vi "Schedule.EditFormula.vi"(8 "error in (no error)":errorcluster, 10 "Settings":string, 11 "ObjectSettings in":refnum<class "ObjectSettings.lvclass">) -> (0 "error out":errorcluster, 2 "Settings Out":string, 3 "ObjectSettings out":refnum<class "ObjectSettings.lvclass">)   [LabVIEW 2019, in "ObjectSettings.lvclass"]
uses:
  ObjectSettings.lvclass
  <vilib>/gmath/NI_Gmath.lvlib
  subVIs/typedefs/Schedule Types/Schedule--Formula.ctl
panel:
  in  "Resolution (nm)":dbl caption="Numeric"
  in  "OK":bool
  in  "Length (nm)":dbl caption="Numeric"
  out "XY Graph":cluster{"X Values":dbl[], "Y Values":dbl[]}(graph)
  in  "Formula":string
  out "Parse Error":bool
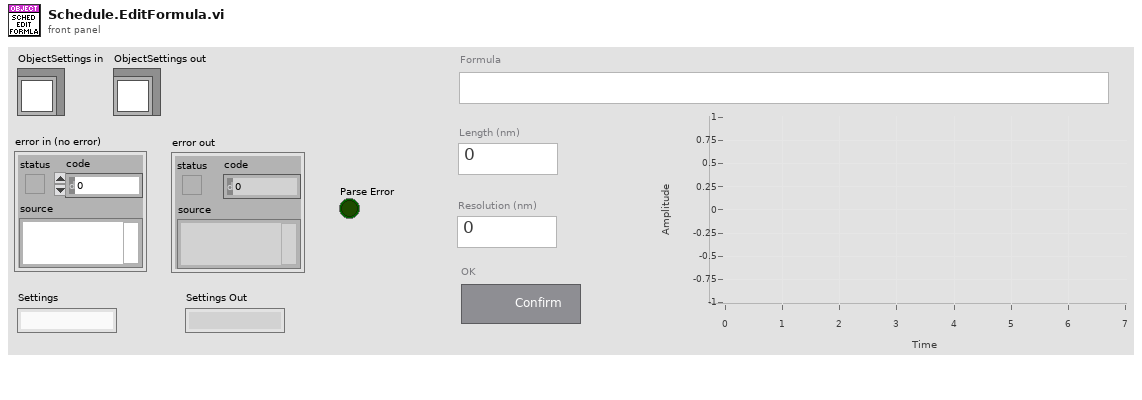
[diagram p1: front panel]
types:
  T1 = enum32{"Invalid", "Standard", "Closed", "Hidden", "Minimized", "Maximized"}
  T2 = enum32{"invalid app kind", "Development System", "Run Time System", "Student Edition", "Embedded LabVIEW", "Evaluation", "Custom"}
  T3 = typedef "Schedule--Formula.ctl" = cluster{"formula":string, "formula length (nm)":dbl, "formula resolution (nm)":dbl}
  T4 = cluster{"Core":cluster{"Current VI Reference":refnum<vi>, "Close Panel on Exit?":bool}, "ObjectSettings":refnum<class "ObjectSettings.lvclass">, "Formula":string, "Length (nm)":dbl, "Resolution (nm)":dbl, "Settings":string}
  T5 = cluster{"Current VI Reference":refnum<vi>, "Close Panel on Exit?":bool}
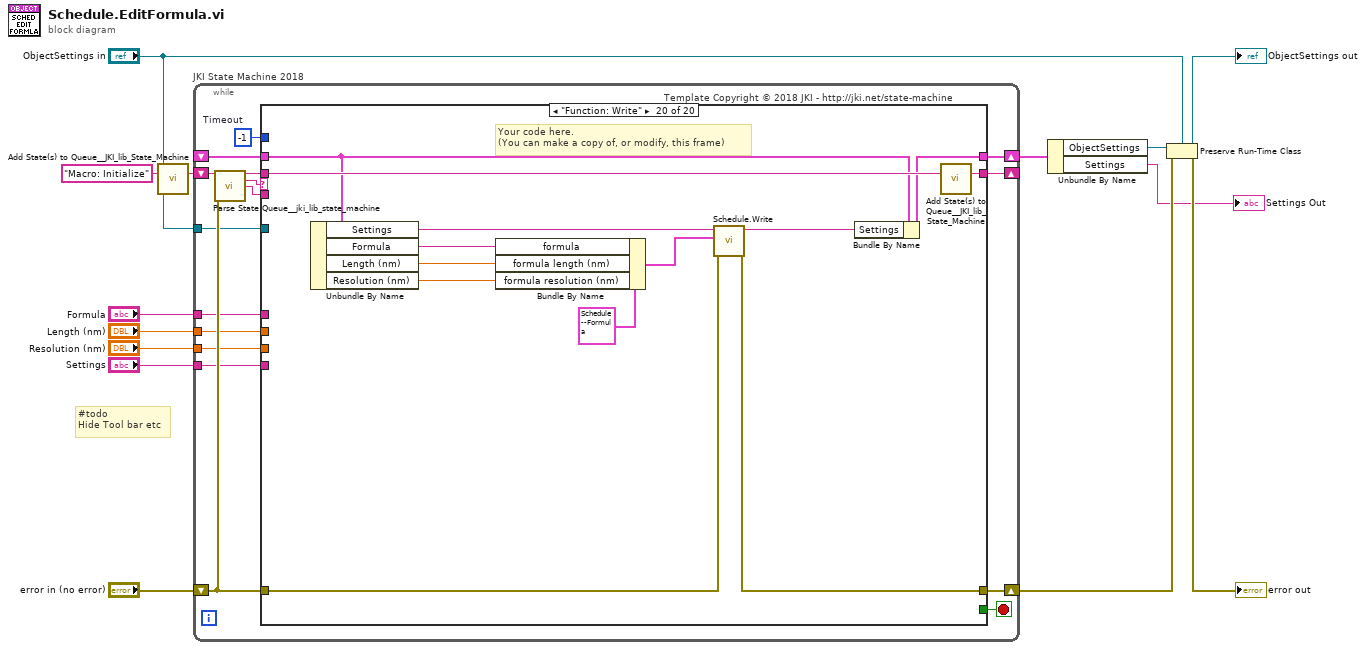
[diagram p0: block diagram]
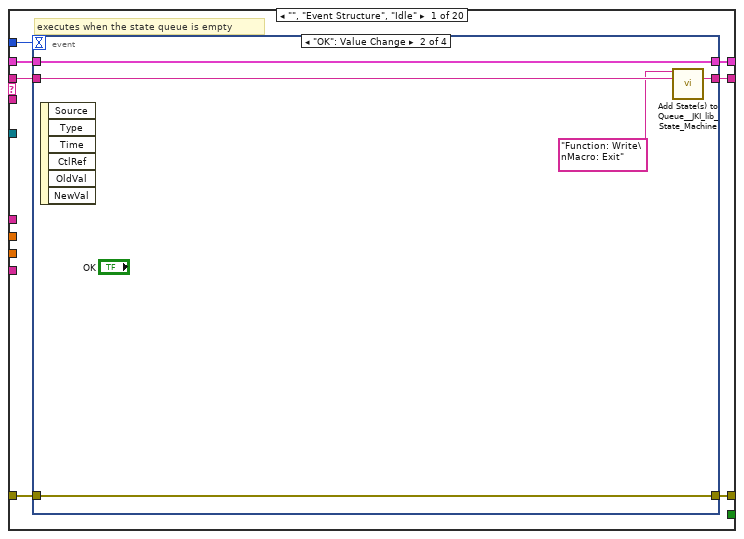
[diagram p2: hidden frame]
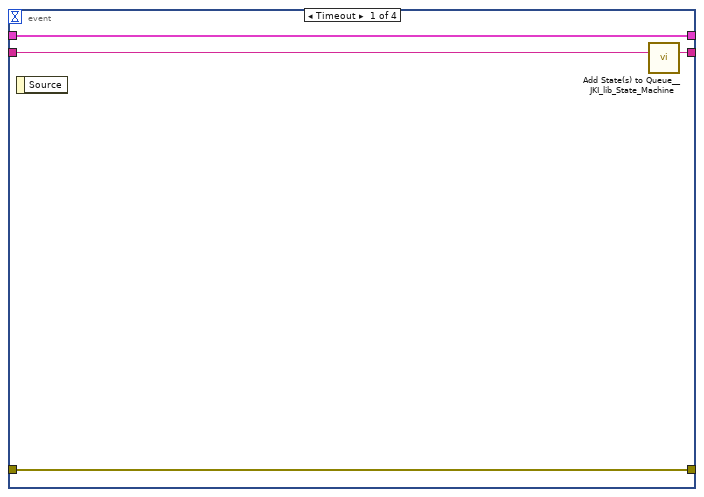
[diagram p3: hidden frame]
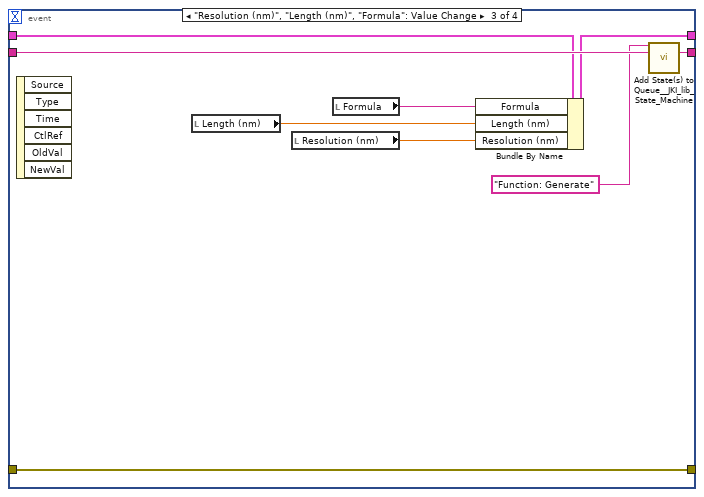
[diagram p4: hidden frame]
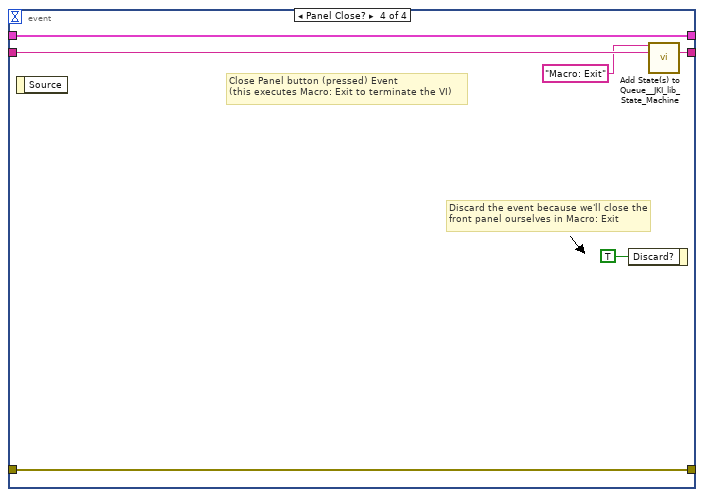
[diagram p5: hidden frame]
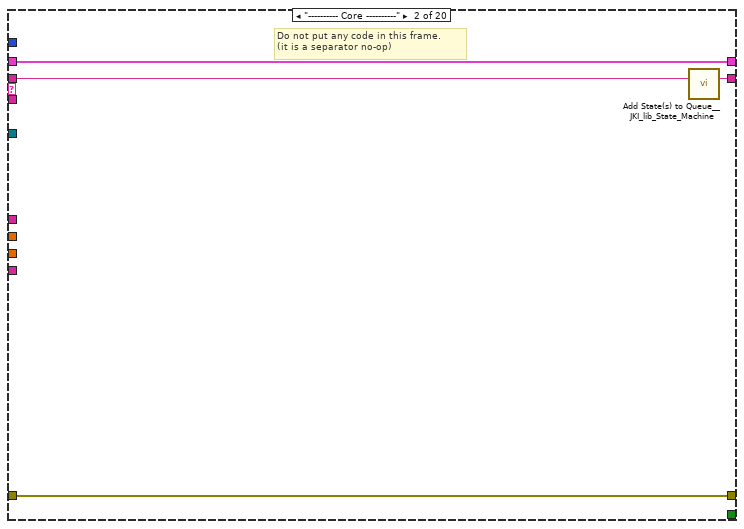
[diagram p6: hidden frame]
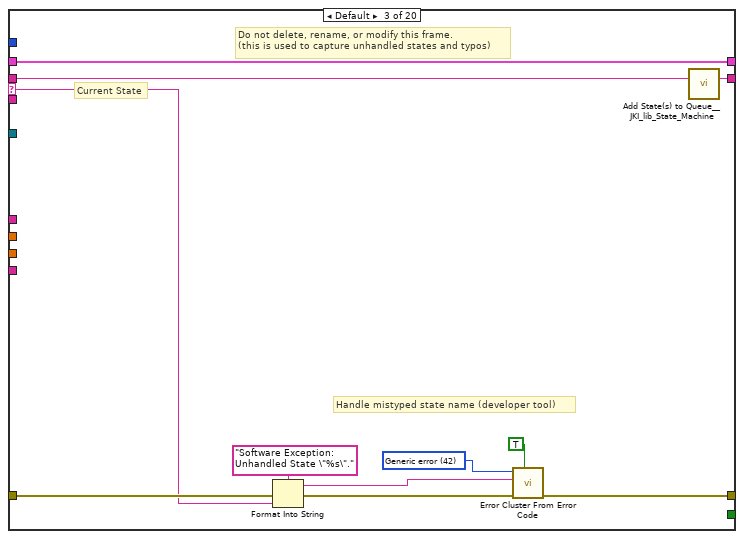
[diagram p7: hidden frame]
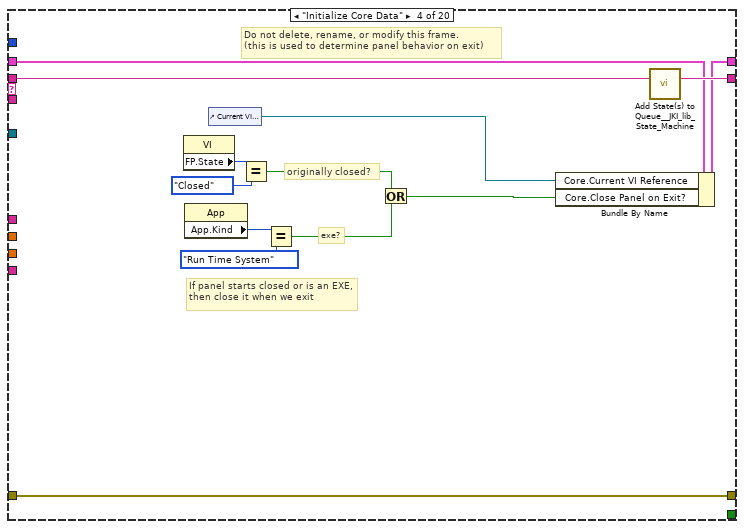
[diagram p8: hidden frame]
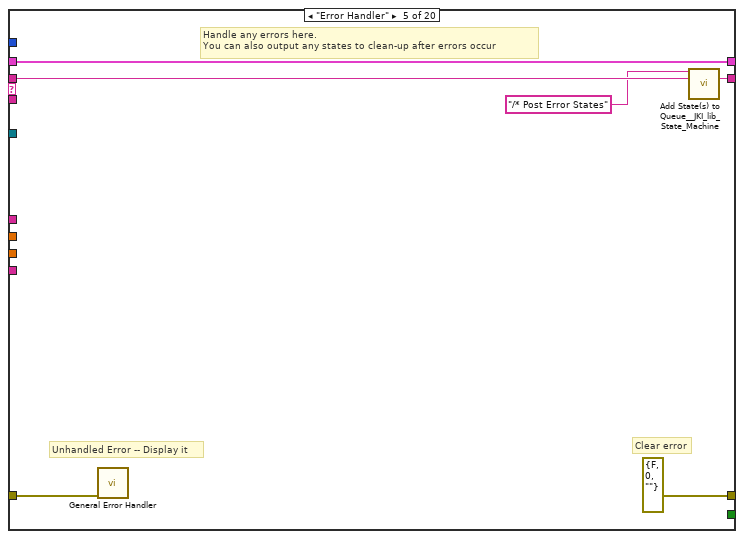
[diagram p9: hidden frame]
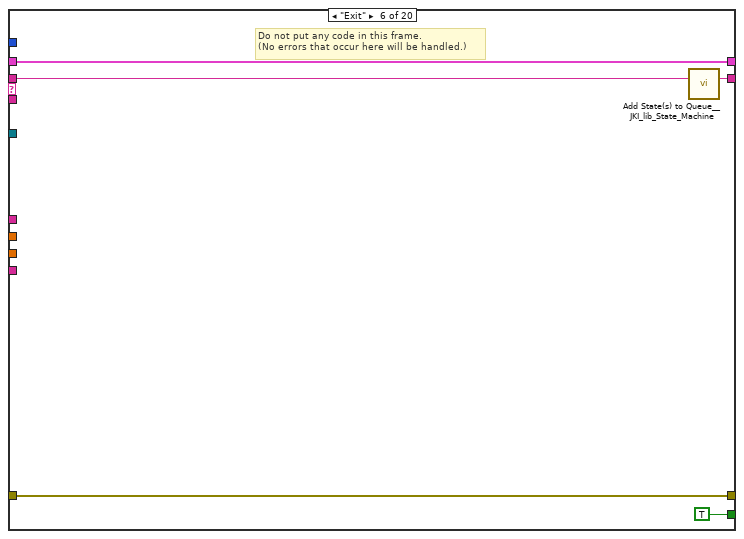
[diagram p10: hidden frame]
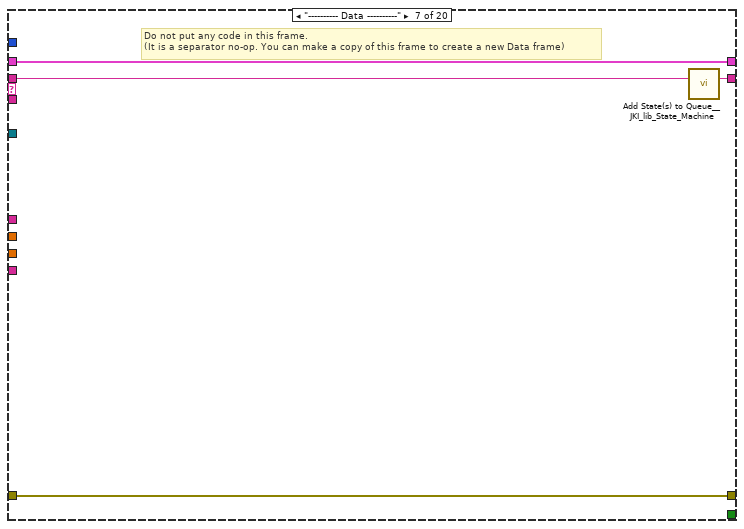
[diagram p11: hidden frame]
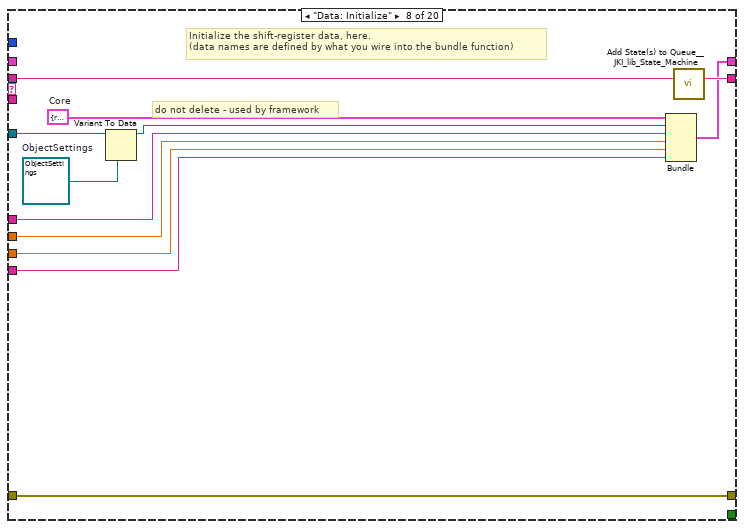
[diagram p12: hidden frame]
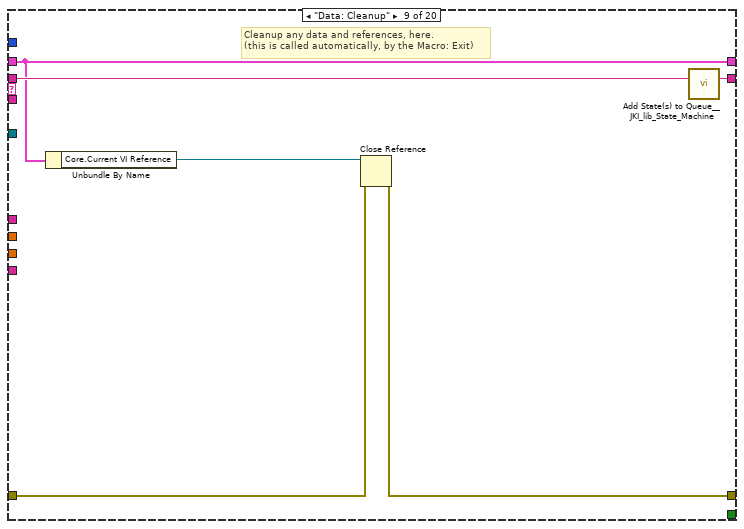
[diagram p13: hidden frame]
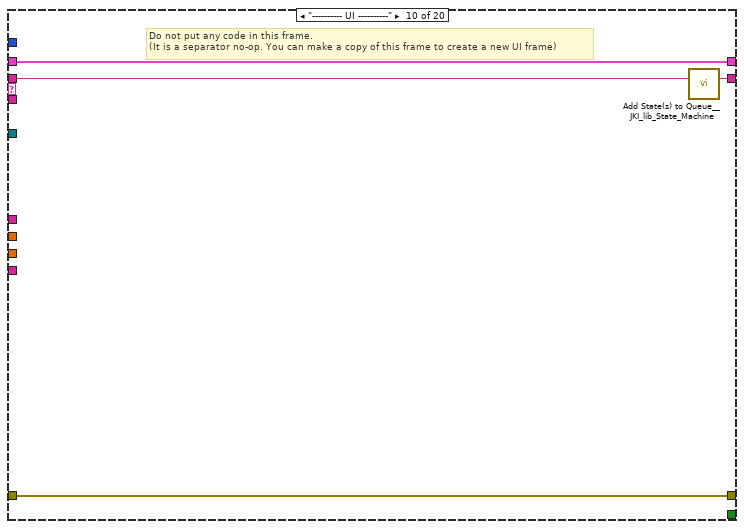
[diagram p14: hidden frame]
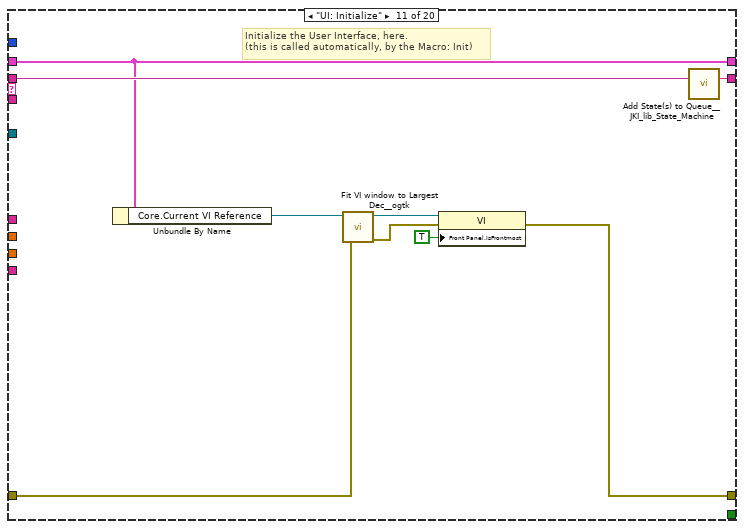
[diagram p15: hidden frame]
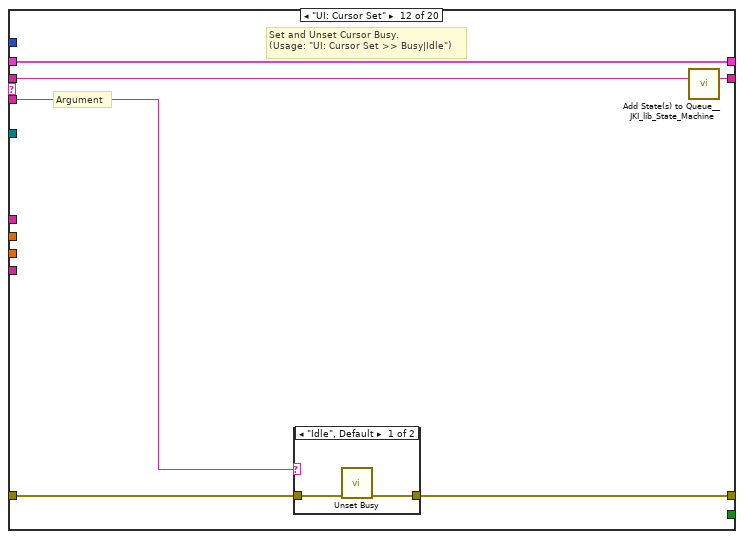
[diagram p16: hidden frame]
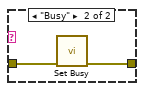
[diagram p17: hidden frame]
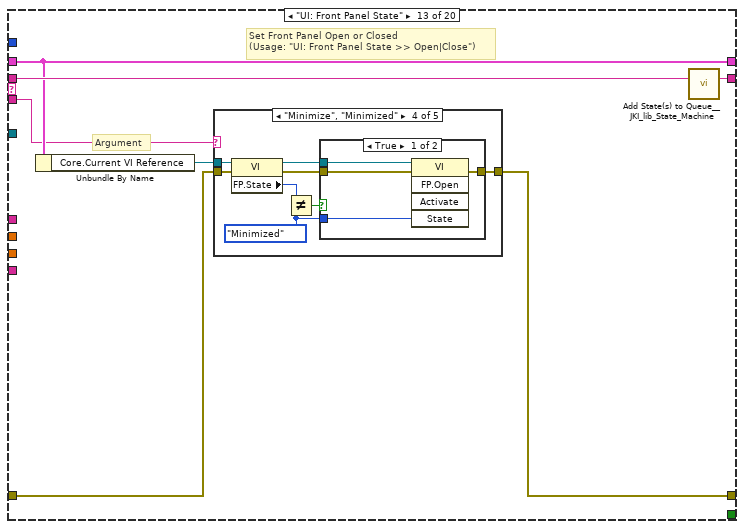
[diagram p18: hidden frame]
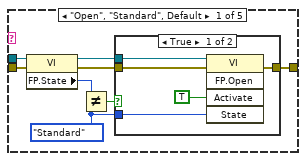
[diagram p19: hidden frame]
diagram:
  # "#todo\nHide Tool bar etc"
  n1 = call <vilib>:"Add State(s) to Queue__JKI_lib_State_Machine.vi"("State(s) in (\"\")"="Macro: Initialize") -> ("States Out"=w14:string)  [unwired: 14 in]
  n2 = while "JKI State Machine 2018" {
    shift-right: [w23] -> w12
    shift-left: _ -> [w22]
    shift-right: [w26] -> w7
    shift-left: "error in (no error)" -> [w20]
    shift-right: [w25] -> _
    shift-left: w14 -> [w27]
    tunnel: "ObjectSettings in" -> [w19]
    tunnel: "Formula" -> [w18]
    tunnel: "Length (nm)" -> [w17]
    tunnel: "Resolution (nm)" -> [w16]
    tunnel: "Settings" -> [w15]
    stop <- w24 stop-if-true
    w21 = -1  # Timeout
    # "Template Copyright © 2018 JKI - http://jki.net/state-machine"
    n3 = call <vilib>:"Parse State Queue__jki_lib_state_machine.vi"("State Queue"=w27, "Error In (no error)"=w20) -> ("Remaining States"=w29:string, "Current State"=w30:string, "Arguments"=w28:string)  [unwired: 11 in]
    n4 = case shown="\"Function: Write\"" w30 {
      selector: w30 -> [_ _ w66 _ _ _ _ _ _ _ _ _ _ _ _ _ _ _ _ _]
      tunnel: w29 -> [w37 w65 w70 w89 w95 w100 w104 w116 w122 w126 w135 w141 w152 w221 w226 w236 w240 w255 w271 w284]
      tunnel: w28 -> [_ _ _ _ _ _ _ _ _ _ _ w136 w146 _ _ _ _ _ _ _]
      tunnel: w22 -> [w35 w62 w68 w82 w92 w98 w101 _ w117 w123 w133 w139 w148 w218 w223 w233 w237 w252 w268 w281]
      tunnel: [w34 w63 w72 w86 errorcluster {"status"=FALSE, "code"=0, "source"=""} ("error out") w97 w102 w113 w118 w124 w127 w137 w149 w219 w224 w234 w238 w242 w269 w272] -> w26
      tunnel: w20 -> [w33 w63 w71 w86 w91 w97 w102 w113 w119 w124 w131 w138 w150 w219 w224 w234 w238 w241 w269 w273]
      tunnel: [w36 w64 w69 w88 w94 w99 w103 w115 w121 w125 w134 w140 w151 w220 w225 w235 w239 w254 w270 w283] -> w25
      tunnel: [_ _ _ _ _ TRUE _ _ _ _ _ _ _ _ _ _ _ _ _ _] -> w24
      tunnel: [w32 w62 w68 w87 w92 w98 w101 w114 w117 w123 w133 w139 w148 w218 w223 w233 w237 w253 w268 w282] -> w23
      tunnel: w21 -> [w31 _ _ _ _ _ _ _ _ _ _ _ _ _ _ _ _ _ _ _]
      tunnel: w19 -> [_ _ _ _ _ _ _ w111 _ _ _ _ _ _ _ _ _ _ _ _]
      tunnel: w18 -> [_ _ _ _ _ _ _ w109 _ _ _ _ _ _ _ _ _ _ _ _]
      tunnel: w17 -> [_ _ _ _ _ _ _ w107 _ _ _ _ _ _ _ _ _ _ _ _]
      tunnel: w16 -> [_ _ _ _ _ _ _ w108 _ _ _ _ _ _ _ _ _ _ _ _]
      tunnel: w15 -> [_ _ _ _ _ _ _ w105 _ _ _ _ _ _ _ _ _ _ _ _]
      frame "", "Event Structure", "Idle" {
        # "executes when the state queue is empty"
        n5 = event shown="[1] \"OK\": Value Change" {
          selector: _ -> [_ _ _ _]
          dyn-events: _ -> [_ _ _ _]
          timeout: w31 -> [_ _ _ _]
          tunnel: w37 -> [w41 w46 w55 w61]
          tunnel: [w40 w45 w54 w60] -> w36
          tunnel: w35 -> [w38 w43 w51 w58]
          tunnel: [w39 w44 w53 w59] -> w34
          tunnel: w33 -> [w39 w44 w53 w59]
          tunnel: [w38 w43 w52 w58] -> w32
          event Timeout {
            n6 = event-data() -> ()  [unwired: 1 in, 1 out]
            n7 = call <vilib>:"Add State(s) to Queue__JKI_lib_State_Machine.vi"("State(s) in (\"\")"=w41) -> ("States Out"=w40:string)  [unwired: 14 in]
          }
          event "OK": Value Change {
            n8 = event-data() -> ()  [unwired: 1 in, 6 out]
            n9 = call <vilib>:"Add State(s) to Queue__JKI_lib_State_Machine.vi"("State(s) in Front (\"\")"="Function: Write\nMacro: Exit", "State(s) in (\"\")"=w46) -> ("States Out"=w45:string)  [unwired: 13 in]
          }
          event "Resolution (nm)", "Length (nm)", "Formula": Value Change {
            n10 = event-data() -> ()  [unwired: 1 in, 6 out]
            n11 = local read "Length (nm)"() -> (w49:dbl)
            n12 = local read "Resolution (nm)"() -> (w50:dbl)
            n13 = local read "Formula"() -> (w48:string)
            n14 = Bundle By Name(cluster=w51, "Formula"=w48, "Length (nm)"=w49, "Resolution (nm)"=w50) -> (w52:T4)
            n15 = call <vilib>:"Add State(s) to Queue__JKI_lib_State_Machine.vi"("State(s) in Front (\"\")"="Function: Generate", "State(s) in (\"\")"=w55) -> ("States Out"=w54:string)  [unwired: 13 in]
          }
          event Panel Close? {
            # "Discard the event because we'll close the front panel ourselves in Macro: Exit"
            # "Close Panel button (pressed) Event\n(this executes Macro: Exit to terminate the VI)"
            n16 = event-data() -> ()  [unwired: 1 in, 1 out]
            n17 = event-data("Discard?"=TRUE) -> ()  [unwired: 1 in, 1 out]
            n18 = call <vilib>:"Add State(s) to Queue__JKI_lib_State_Machine.vi"("State(s) in Front (\"\")"="Macro: Exit", "State(s) in (\"\")"=w61) -> ("States Out"=w60:string)  [unwired: 13 in]
          }
        }
      }
      frame "---------- Core ----------" {
        # "Do not put any code in this frame.\n(it is a separator no-op)"
        n19 = call <vilib>:"Add State(s) to Queue__JKI_lib_State_Machine.vi"("State(s) in (\"\")"=w65) -> ("States Out"=w64:string)  [unwired: 14 in]
      }
      frame Default {
        w75 = 42 items=["No error", "Argument error", "Memory is full", "Out of zone", "End of file", "File already open", "Generic file I/O error", "File not found", "File permission error", "Disk is full", "Duplicate path", "Too many files open", "System feature not enabled", "Resource file not found", "Cannot add resource", "Resource not found", "Image not found", "Image memory error", "Pen does not exist", "Config type invalid", "Config token not found", "Config parse error", "Config memory error", "Bad external code format", "Bad external code offset", "External code not present", "Null window", "Destroy window error", "Null menu", "Print aborted", "Bad print record", "Print driver error", "Windows error during printing", "Memory error during printing", "Print dialog error", "Generic print error", "Invalid device refnum", "Device not found", "Device parameter error", "Device unit error", "Cannot open device", "Device call aborted", "Generic error", "Cancelled by user", "Object ID too low", "Object ID too high", "Object not in heap", "Unknown heap", "Unknown object (invalid DefProc)", "Unknown object (DefProc not in table)", "Message out of range", "Invalid (null) method", "Unknown message", "Manager call not supported", "Bad address", "Network operation in progress", "Network operation timed out", "Connection is busy", "Network attribute not supported", "Network error", "Address in use", "System out of memory", "Connection aborted", "Connection refused", "Not connected", "Already connected", "Connection closed", "Initialization error (interapplication manager)", "Bad occurrence", "Wait on unbound occurrence handler", "Occurrence queue overflow", "Datalog type conflict", "Unused", "Unrecognized type (interapplication manager)", "Memory corrupt", "Failed to make temporary DLL", "Old CIN version", "Drag socket not found", "Failed to load drop-object", "Failed to register OLE object", "Failed to release OLE object", "Format specifier type mismatch", "Unknown format specifier", "Too few format specifiers", "Too many format specifiers", "Scan failed", "Newer CIN version", "Error converting to variant", "Runtime menu error", "Password tampered", "Variant attribute not found", "Incompatible variant data type", "Event data is not available", "Event Store is not present", "Occurrence is not found", "Event Queue is not created", "Event info is not available", "Refnum passed is NULL", "Error retrieving Class GUID", "Error retrieving CoClass GUID", "Error retrieving TypeLib GUID.", "Bad built application magic bytes.", "Specific driver is different from the specific driver associated with the Logical Name.", "There is no session opened to the class driver.", "Max Error", "MAX - Error with config objects", "MAX - Error loading configuration", "MAX - Group not supported"]
        # "Current State"
        # "Do not delete, rename, or modify this frame.\n(this is used to capture unhandled states and typos)"
        # "Handle mistyped state name (developer tool)"
        n20 = Format Into String(format string="Software Exception: Unhandled State \"%s\"." ("message"), error in=w71, w66) -> (resulting string=w74:string, error out=w73:errorcluster)  [unwired: 1 in]
        n21 = call <vilib>:"Error Cluster From Error Code.vi"("show call chain? (False)"=TRUE, "error in (no error)"=w73, "error message (\"\")"=w74, "error code (0)"=w75) -> ("error out"=w72:errorcluster)  [unwired: 5 in]
        n22 = call <vilib>:"Add State(s) to Queue__JKI_lib_State_Machine.vi"("State(s) in (\"\")"=w70) -> ("States Out"=w69:string)  [unwired: 14 in]
      }
      frame "Initialize Core Data" {
        # "Do not delete, rename, or modify this frame.\n(this is used to determine panel behavior on exit)"
        # "originally closed?"
        # "exe?"
        # "If panel starts closed or is an EXE, then close it when we exit"
        n23 = property class="VI"() -> ("FP.State"=w79:T1)  [unwired: 2 in, 2 out]
        n24 = property class="App"() -> ("App.Kind"=w85:T2)  [unwired: 2 in, 2 out]
        n25 = control-ref of="Current VI Reference"() -> (w80:refnum<vi>)
        n26 = Equal?(x=w79, y=T1."Closed" ("Front Panel Window:State")) -> (x = y?=w77:bool)
        n27 = Equal?(x=w85, y=T2."Run Time System" ("Application:Kind")) -> (x = y?=w83:bool)
        n28 = Or(x=w77, y=w83) -> (x .or. y?=w81:bool)
        n29 = Bundle By Name(cluster=w82, "Core.Current VI Reference"=w80, "Core.Close Panel on Exit?"=w81) -> (w87:T4)
        n30 = call <vilib>:"Add State(s) to Queue__JKI_lib_State_Machine.vi"("State(s) in (\"\")"=w89) -> ("States Out"=w88:string)  [unwired: 14 in]
      }
      frame "Error Handler" {
        # "Unhandled Error -- Display it"
        # "Handle any errors here.\nYou can also output any states to clean-up after errors occur"
        # "Clear error"
        n31 = call <vilib>:"General Error Handler.vi"("error in (no error)"=w91) -> ()  [unwired: 10 in, 5 out]
        n32 = call <vilib>:"Add State(s) to Queue__JKI_lib_State_Machine.vi"("State(s) in Front (\"\")"="/* Post Error States", "State(s) in (\"\")"=w95) -> ("States Out"=w94:string)  [unwired: 13 in]
      }
      frame "Exit" {
        # "Do not put any code in this frame.\n(No errors that occur here will be handled.)"
        n33 = call <vilib>:"Add State(s) to Queue__JKI_lib_State_Machine.vi"("State(s) in (\"\")"=w100) -> ("States Out"=w99:string)  [unwired: 14 in]
      }
      frame "---------- Data ----------" {
        # "Do not put any code in this frame.\n(It is a separator no-op. You can make a copy of this frame to create a new Data frame)"
        n34 = call <vilib>:"Add State(s) to Queue__JKI_lib_State_Machine.vi"("State(s) in (\"\")"=w104) -> ("States Out"=w103:string)  [unwired: 14 in]
      }
      frame "Data: Initialize" {
        w110 = refnum<class "ObjectSettings.lvclass"> refnum  # ObjectSettings
        w112 = T5 {"Current VI Reference"=refnum, "Close Panel on Exit?"=FALSE}  # Core
        # "do not delete - used by framework"
        # "Initialize the shift-register data, here.\n(data names are defined by what you wire into the bundle function)"
        n35 = Variant To Data(type=w110, Variant=w111) -> (data=w106:refnum<class "ObjectSettings.lvclass">)  [unwired: 1 in, 1 out]
        n36 = Bundle("Core"=w112, "ObjectSettings"=w106, "Formula"=w109, "Length (nm)"=w107, "Resolution (nm)"=w108, "Settings"=w105) -> (w114:T4)  [unwired: 1 in]
        n37 = call <vilib>:"Add State(s) to Queue__JKI_lib_State_Machine.vi"("State(s) in (\"\")"=w116) -> ("States Out"=w115:string)  [unwired: 14 in]
      }
      frame "Data: Cleanup" {
        # "Cleanup any data and references, here.\n(this is called automatically, by the Macro: Exit)"
        n38 = Unbundle By Name(w117) -> ("Core.Current VI Reference"=w120:refnum<vi>)
        n39 = Close Reference(reference=w120, error in (no error)=w119) -> (error out=w118:errorcluster)
        n40 = call <vilib>:"Add State(s) to Queue__JKI_lib_State_Machine.vi"("State(s) in (\"\")"=w122) -> ("States Out"=w121:string)  [unwired: 14 in]
      }
      frame "---------- UI ----------" {
        # "Do not put any code in this frame.\n(It is a separator no-op. You can make a copy of this frame to create a new UI frame)"
        n41 = call <vilib>:"Add State(s) to Queue__JKI_lib_State_Machine.vi"("State(s) in (\"\")"=w126) -> ("States Out"=w125:string)  [unwired: 14 in]
      }
      frame "UI: Initialize" {
        # "Initialize the User Interface, here.\n(this is called automatically, by the Macro: Init)"
        n42 = Unbundle By Name(w133) -> ("Core.Current VI Reference"=w132:refnum<vi>)
        n43 = call <userlib>:"Fit VI window to Largest Dec__ogtk.vi"("error in (no error)"=w131, "VI Ref (calling VI)"=w132) -> ("error out"=w128:errorcluster, "dup VI Ref"=w130:refnum<vi>)  [unwired: 4 in]
        n44 = property class="VI"(reference=w130, error in=w128, "Front Panel.IsFrontmost"=TRUE ("Front Panel Window:Is Frontmost")) -> (error out=w127:errorcluster)  [unwired: 1 out]
        n45 = call <vilib>:"Add State(s) to Queue__JKI_lib_State_Machine.vi"("State(s) in (\"\")"=w135) -> ("States Out"=w134:string)  [unwired: 14 in]
      }
      frame "UI: Cursor Set" {
        # "Argument"
        # "Set and Unset Cursor Busy.\n(Usage: \"UI: Cursor Set >> Busy|Idle\")"
        n46 = case shown="\"Idle\", Default" w136 {
          tunnel: w138 -> [w143 w145]
          tunnel: [w142 w144] -> w137
          frame "Idle", Default {
            n47 = call <vilib>:"Unset Busy.vi"("error in (no error)"=w143) -> ("error out"=w142:errorcluster)  [unwired: 10 in]
          }
          frame "Busy" {
            n48 = call <vilib>:"Set Busy.vi"("error in (no error)"=w145) -> ("error out"=w144:errorcluster)  [unwired: 9 in, 1 out]
          }
        }
        n49 = call <vilib>:"Add State(s) to Queue__JKI_lib_State_Machine.vi"("State(s) in (\"\")"=w141) -> ("States Out"=w140:string)  [unwired: 14 in]
      }
      frame "UI: Front Panel State" {
        # "Argument"
        # "Set Front Panel Open or Closed\n(Usage: \"UI: Front Panel State >> Open|Close\")"
        n50 = Unbundle By Name(w148) -> ("Core.Current VI Reference"=w147:refnum<vi>)
        n51 = case shown="\"Minimize\", \"Minimized\"" w146 {
          tunnel: w150 -> [w158 w173 w184 w197 w210]
          tunnel: [w160 w174 w186 w199 w212] -> w149
          tunnel: w147 -> [w159 w171 w185 w198 w211]
          frame "Open", "Standard", Default {
            w153 = T1."Standard" ("State")
            n52 = property class="VI"(reference=w159, error in=w158) -> (reference out=w156:refnum<vi>, error out=w157:errorcluster, "FP.State"=w155:T1)
            n53 = Not Equal?(x=w155, y=w153) -> (x != y?=w154:bool)
            n54 = case shown="True" w154 {
              tunnel: [w164 w166] -> w160
              tunnel: w157 -> [w163 w166]
              tunnel: w156 -> [w162 _]
              tunnel: w153 -> [w161 _]
              frame True {
                n55 = invoke class="VI" method="FP.Open"(reference=w162, error in=w163, "Activate"=TRUE, "State"=w161) -> (error out=w164:errorcluster)  [unwired: 1 in, 4 out]
              }
              frame False {
              }
            }
          }
          frame "Close", "Closed" {
            n56 = property class="VI"(reference=w171, error in=w173) -> (reference out=w170:refnum<vi>, error out=w172:errorcluster, "FP.State"=w168:T1)
            n57 = Not Equal?(x=w168, y=T1."Closed" ("Front Panel Window:State")) -> (x != y?=w167:bool)
            n58 = case shown="True" w167 {
              tunnel: [w175 w178] -> w174
              tunnel: w172 -> [w175 w177]
              tunnel: w170 -> [_ w176]
              frame False {
              }
              frame True {
                n59 = invoke class="VI" method="FP.Close"(reference=w176, error in=w177) -> (error out=w178:errorcluster)  [unwired: 1 in, 2 out]
              }
            }
          }
          frame "Hidden", "Hide" {
            w179 = T1."Hidden" ("State")
            n60 = property class="VI"(reference=w185, error in=w184) -> (reference out=w182:refnum<vi>, error out=w183:errorcluster, "FP.State"=w181:T1)
            n61 = Not Equal?(x=w181, y=w179) -> (x != y?=w180:bool)
            n62 = case shown="True" w180 {
              tunnel: [w190 w191] -> w186
              tunnel: w183 -> [w189 w191]
              tunnel: w182 -> [w188 _]
              tunnel: w179 -> [w187 _]
              frame True {
                n63 = invoke class="VI" method="FP.Open"(reference=w188, error in=w189, "State"=w187) -> (error out=w190:errorcluster)  [unwired: 2 in, 4 out]
              }
              frame False {
              }
            }
          }
          frame "Minimize", "Minimized" {
            w192 = T1."Minimized" ("State")
            n64 = property class="VI"(reference=w198, error in=w197) -> (reference out=w195:refnum<vi>, error out=w196:errorcluster, "FP.State"=w194:T1)
            n65 = Not Equal?(x=w194, y=w192) -> (x != y?=w193:bool)
            n66 = case shown="True" w193 {
              tunnel: [w203 w204] -> w199
              tunnel: w196 -> [w202 w204]
              tunnel: w195 -> [w201 _]
              tunnel: w192 -> [w200 _]
              frame True {
                n67 = invoke class="VI" method="FP.Open"(reference=w201, error in=w202, "State"=w200) -> (error out=w203:errorcluster)  [unwired: 2 in, 4 out]
              }
              frame False {
              }
            }
          }
          frame "Maximize", "Maximized" {
            w205 = T1."Maximized" ("State")
            n68 = property class="VI"(reference=w211, error in=w210) -> (reference out=w208:refnum<vi>, error out=w209:errorcluster, "FP.State"=w207:T1)
            n69 = Not Equal?(x=w207, y=w205) -> (x != y?=w206:bool)
            n70 = case shown="True" w206 {
              tunnel: [w216 w217] -> w212
              tunnel: w209 -> [w215 w217]
              tunnel: w208 -> [w214 _]
              tunnel: w205 -> [w213 _]
              frame True {
                n71 = invoke class="VI" method="FP.Open"(reference=w214, error in=w215, "State"=w213) -> (error out=w216:errorcluster)  [unwired: 2 in, 4 out]
              }
              frame False {
              }
            }
          }
        }
        n72 = call <vilib>:"Add State(s) to Queue__JKI_lib_State_Machine.vi"("State(s) in (\"\")"=w152) -> ("States Out"=w151:string)  [unwired: 14 in]
      }
      frame "---------- Macro ----------" {
        # "Do not put any code in this frame.\n(It is a separator no-op. You can make a copy of this frame to create a new Macro frame)"
        n73 = call <vilib>:"Add State(s) to Queue__JKI_lib_State_Machine.vi"("State(s) in (\"\")"=w221) -> ("States Out"=w220:string)  [unwired: 14 in]
      }
      frame "Macro: Initialize" {
        w222 = "Data: Initialize\nInitialize Core Data\nFunction: Read\nUI: Initialize\nUI: Front Panel State >> Open"  # Data: Initialize Initialize Core Data Function: Read UI: Initialize UI: Front Panel State >> Open
        # "Initialization Macro\n(This is called once, when the VI starts)"
        n74 = call <vilib>:"Add State(s) to Queue__JKI_lib_State_Machine.vi"("State(s) in Front (\"\")"=w222, "State(s) in (\"\")"=w226) -> ("States Out"=w225:string)  [unwired: 13 in]
      }
      frame "Macro: Exit" {
        # "Exit Macro\n(This is called once, when the VI exits)"
        n75 = Unbundle By Name(w233) -> ("Core.Close Panel on Exit?"=w232:bool)
        n76 = Select(t="UI: Front Panel State >> Close", s=w232, f="") -> (s? t:f=w229:string)
        n77 = call <vilib>:"Add State(s) to Queue__JKI_lib_State_Machine.vi"("State(s) in (\"\")"=w229, "State(s) at Back (\"\")"="Data: Cleanup\nExit") -> ("States Out"=w227:string)  [unwired: 13 in]
        n78 = call <vilib>:"Add State(s) to Queue__JKI_lib_State_Machine.vi"("State(s) in Front (\"\")"=w227, "State(s) in (\"\")"=w236) -> ("States Out"=w235:string)  [unwired: 13 in]
      }
      frame "---------- Function ----------" {
        # "Template Separator\n(You can make a copy of, or modify, this frame)"
        n79 = call <vilib>:"Add State(s) to Queue__JKI_lib_State_Machine.vi"("State(s) in (\"\")"=w240) -> ("States Out"=w239:string)  [unwired: 14 in]
      }
      frame "Function: Read" {
        w244 = T3 {"formula"="1*(step(170-t)*cos(0.62831853071*t)+step(t-170)*cos(0.62831853071*(t-170))*(-1))", "formula length (nm)"=1.0, "formula resolution (nm)"=0.001} ("Formula")
        # "Template Separator\n(You can make a copy of, or modify, this frame)"
        n80 = Unbundle By Name(w252) -> ("Settings"=w247:string)
        n81 = call "Schedule.Read.vi"("Data to Read"=w244, "error in (no error)"=w241, "Schedule <JSON> In"=w247) -> ("error out"=w243:errorcluster, "Data Out"=w245:variant, "Schedule <JSON> Out"=w246:string)  [unwired: 6 in]
        n82 = Variant To Data(error in=w243, type=w244, Variant=w245) -> (data=w248:T3, error out=w242:errorcluster)
        n83 = Unbundle By Name(w248) -> ("formula"=w251:string, "formula length (nm)"=w250:dbl, "formula resolution (nm)"=w249:dbl)
        n84 = Bundle By Name(cluster=w252, "Settings"=w246, "Formula"=w251, "Length (nm)"=w250, "Resolution (nm)"=w249) -> (w253:T4)
        n85 = local write "Resolution (nm)"(w249) -> ()
        n86 = local write "Length (nm)"(w250) -> ()
        n87 = local write "Formula"(w251) -> ()
        n88 = call <vilib>:"Add State(s) to Queue__JKI_lib_State_Machine.vi"("State(s) in (\"\")"=w255) -> ("States Out"=w254:string)  [unwired: 14 in]
      }
      frame "Function: Generate" {
        # "Your code here.\n(You can make a copy of, or modify, this frame)"
        n89 = Unbundle By Name(w268) -> ("Length (nm)"=w267:dbl, "Resolution (nm)"=w266:dbl, "Formula"=w257:string)
        n90 = call "Formula Replace Pi.vi"("Formula In"=w257) -> ("Formula Out"=w256:string)  [unwired: 4 in]
        n91 = Divide(x=w267, y=w266) -> (x/y=w265:dbl)
        n92 = To Unsigned Long Integer(number=w265) -> (unsigned 32bit integer=w263:u32)
        n93 = call <vilib>:"Eval y=f(x).vi"("formula"=w256, "end"=w267, "start"=0.0, "number of points"=w263) -> ("error"=w260:i32, "Y Values"=w261:dbl[], "X Values"=w262:dbl[])  [unwired: 1 out]
        n94 = Bundle("X Values"=w262, "Y Values"=w261) -> (→"XY Graph":cluster{"X Values":dbl[], "Y Values":dbl[]})  [unwired: 1 in]
        n95 = Not Equal To 0?(x=w260) -> (x != 0?=→"Parse Error":bool)
        n96 = call <vilib>:"Add State(s) to Queue__JKI_lib_State_Machine.vi"("State(s) in (\"\")"=w271) -> ("States Out"=w270:string)  [unwired: 14 in]
      }
      frame "Function: Write" {
        # "Your code here.\n(You can make a copy of, or modify, this frame)"
        n97 = Unbundle By Name(w281) -> ("Settings"=w276:string, "Formula"=w279:string, "Length (nm)"=w278:dbl, "Resolution (nm)"=w277:dbl)
        n98 = Bundle By Name(cluster=T3 {"formula"="1*(step(170-t)*cos(0.62831853071*t)+step(t-170)*cos(0.62831853071*(t-170))*(-1))", "formula length (nm)"=340.0, "formula resolution (nm)"=0.001} ("Formula"), "formula"=w279, "formula length (nm)"=w278, "formula resolution (nm)"=w277) -> (w274:T3)
        n99 = call "Schedule.Write.vi"("error in (no error)"=w273, "Data to Write"=w274, "Schedule <JSON> In"=w276) -> ("error out"=w272:errorcluster, "Schedule <JSON> Out"=w275:string)  [unwired: 7 in]
        n100 = Bundle By Name(cluster=w281, "Settings"=w275) -> (w282:T4)
        n101 = call <vilib>:"Add State(s) to Queue__JKI_lib_State_Machine.vi"("State(s) in (\"\")"=w284) -> ("States Out"=w283:string)  [unwired: 14 in]
      }
    }
  }
  n102 = Unbundle By Name(w12) -> ("ObjectSettings"=w10:refnum<class "ObjectSettings.lvclass">, "Settings"=→"Settings Out":string)
  n103 = Preserve Run-Time Class(object in=w10, error in=w7, 2:"ObjectSettings in") -> (object out=→"ObjectSettings out":refnum<class "ObjectSettings.lvclass">, error out=→"error out":errorcluster)
